vi "VI Server_GenerateTabControlList.vi"(8 "error in (no error)":errorcluster, 11 "VI Server Cluster":T1) -> (0 "error out":errorcluster, 3 "VI Server Cluster.DUP":T1, 5 "TabControls":string[](array[string]))   [LabVIEW 2020, in "VI Server Toolkit LV2013.lvlib"]
doc: "Generates a list of Tab Controls."
uses:
  VI Server Toolkit LV2013.lvlib
  VI Server_TypeDefs/VI Server_RefsCluster.ctl
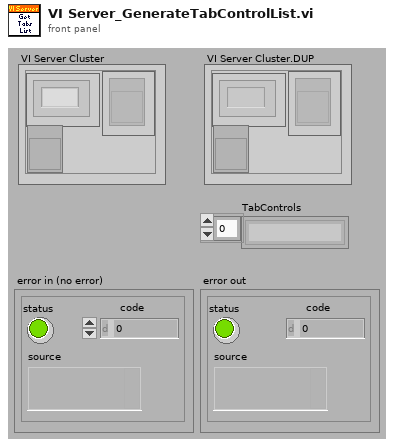
[diagram p1: front panel]
types:
  T1 = typedef "VI Server_RefsCluster.ctl" = cluster{"Labels":string[], "Refs":refnum<vi>[], "VI Ref":refnum<vi>}
  T2 = typedef "VI Server Toolkit LV2013.lvlib/VI Server_DataType.ctl" = enum16{"", "Digital [Dbl]", "Digital [Sgl]", "Digital [I32]", "Digital [I16]", "Digital [I8]", "Digital [U32]", "Digital [U16]", "Digital [U8]", "Boolean", "Slide [Dbl]", "Slide [Sgl]", "Slide [I32]", "Slide [I16]", "Slide [I8]", "Slide [U32]", "Slide [U16]", "Slide [U8]", "Enumerated", "Path", "VISA Resource Name", "Text Ring", "String", "TabControl", "Knob [U8]", "Knob [U16]", "Knob [U32]", "Knob [I8]", "Knob [I16]", "Knob [I32]", "Knob [SGL]", "Knob [DBL]"}
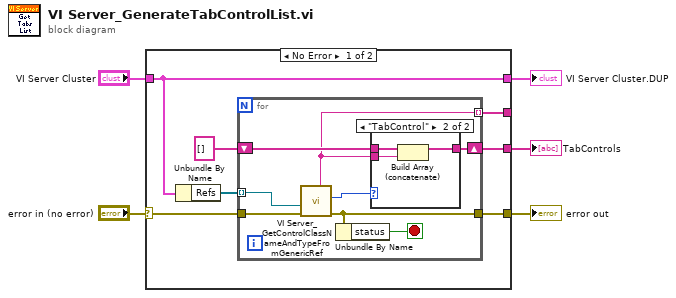
[diagram p0: block diagram]
diagram:
  n1 = case shown="No Error" "error in (no error)" {
    selector: "error in (no error)" -> [w11 w25]
    tunnel: [w9 w25] -> w5
    tunnel: "VI Server Cluster" -> [w12 _]
    tunnel: [w12 _] -> w2
    tunnel: [w7 _] -> w1
    tunnel: [w6 _] -> _
    frame No Error {
      n2 = Unbundle By Name(w12) -> ("Refs"=w10:refnum<vi>[])
      n3 = for {
        tunnel: w11 -> [w20]
        tunnel: w10 -> [w19] mode=indexing
        tunnel: [w15] -> w9
        shift-right: [w16] -> w7
        shift-left: string[] [] -> [w17]
        tunnel: [w13] -> w6 mode=indexing
        stop <- w14 stop-if-true
        n4 = call "VI Server_GetControlClassNameAndTypeFromGenericRef.vi"("error in (no error)"=w20, "Control Reference"=w19) -> ("error out"=w15:errorcluster, "ControlType"=w18:T2, "ControlLabel"=w13:string)  [unwired: 6 in, 1 out]
        n5 = Unbundle By Name(w15) -> ("status"=w14:bool)
        n6 = case shown="\"TabControl\"" w18 {
          tunnel: w17 -> [w21 w24]
          tunnel: w13 -> [_ w23]
          tunnel: [w21 w22] -> w16
          frame "", Default {
          }
          frame "TabControl" {
            n7 = Build Array (concatenate)(w24, w23) -> (w22:string[])
          }
        }
      }
    }
    frame Error {
    }
  }
  "error out" <- w5
  "VI Server Cluster.DUP" <- w2
  "TabControls" <- w1
